vi "Advanced Generate LV Icon.vi"() -> ()   [LabVIEW 2020, in "LabVIEW Icon API.lvlib"]
doc: "This example shows an advanced way of using the LabVIEW Icon API."
uses:
  LabVIEW Icon API.lvlib
  lv_icon/Classes/Icon/Icon.lvclass
  API_Rectangle Dimension.ctl
  API_Text.ctl
  <vilib>/picture/picture.llb/imagedata.ctl
  <vilib>/Utility/miscctls.llb/LVPoint32TypeDef.ctl
  API_User Layer Data.ctl
  <vilib>/Utility/miscctls.llb/LVRectTypeDef.ctl
  API_Rectangle Colors.ctl
panel:
  out "Library Icon applied VI Icon":picture
  out "Updated VI Icon":picture
  out "Original VI Icon":picture
  out "Updated Library Icon":picture
  out "Original Library Icon":picture
  in  "Layer name":string="Circle"
  out "error out":errorcluster
  in  "error in (no error)":errorcluster
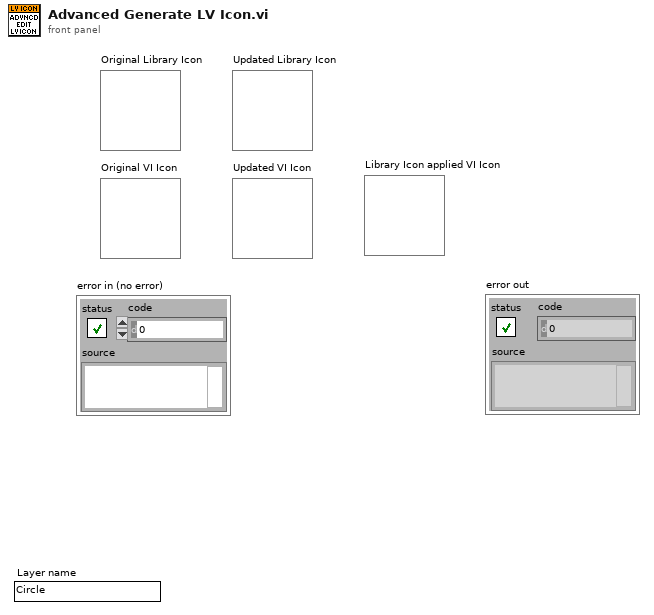
[diagram p1: front panel]
types:
  T1 = typedef "LabVIEW Icon API.lvlib/API_Rectangle Colors.ctl" = cluster{"Border":u32, "Background":u32}
  T2 = typedef "LVRectTypeDef.ctl" = cluster{"Left":i16, "Top":i16, "Right":i16, "Bottom":i16}
  T3 = cluster{"left":i16, "top":i16, "right":i16, "bottom":i16}
  T4 = typedef "LabVIEW Icon API.lvlib/API_User Layer Data.ctl" = cluster{"Layer name":string, "Origin":T5, "Icon image data":T6}
  T5 = typedef "LVPoint32TypeDef.ctl" = cluster{"Horizontal":i32, "Vertical":i32}
  T6 = typedef "imagedata.ctl" = cluster{"image type":i32, "image depth":i32, "image":u8[], "mask":u8[], "colors":u32[], "Rectangle":cluster{"left":i16, "top":i16, "right":i16, "bottom":i16}}
  T7 = typedef "LabVIEW Icon API.lvlib/API_Text.ctl" = cluster{"Line 1 text":string, "Line 2 text":string, "Line 3 text":string, "Line 4 text":string}
  T8 = typedef "LabVIEW Icon API.lvlib/API_Rectangle Dimension.ctl" = cluster{"Width":i16, "Height":i16}
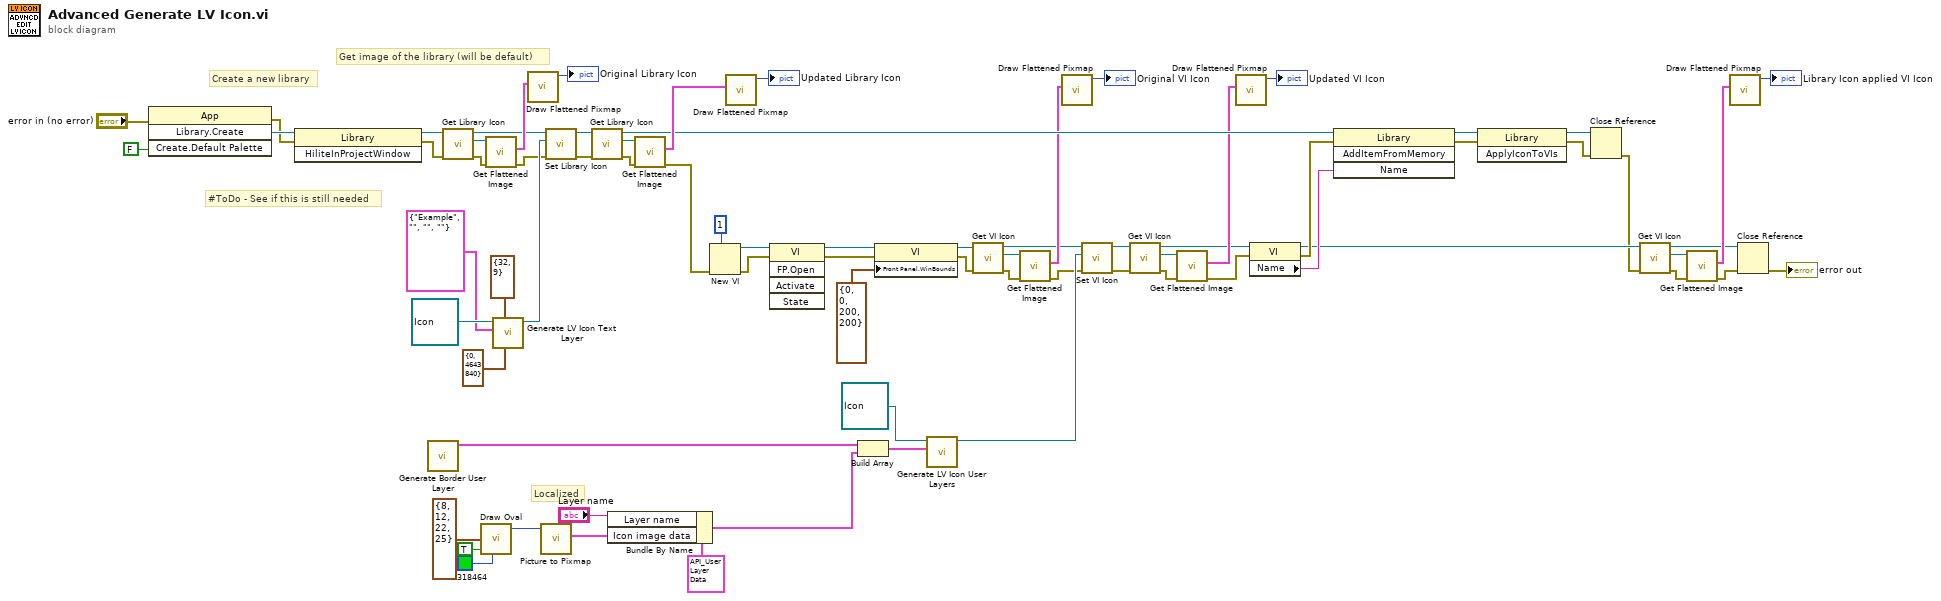
[diagram p0: block diagram]
diagram:
  # "#ToDo - See if this is still needed"
  # "Create a new library"
  # "Get image of the library (will be default)"
  # "Localized"
  n1 = invoke class="App" method="Library.Create"(error in="error in (no error)", "Create.Default Palette"=FALSE ("Create:Default Palette")) -> (error out=w67:errorcluster, "Create Library"=w68:refnum<vi>)  [unwired: 2 in, 2 out]
  n2 = invoke class="Library" method="HiliteInProjectWindow"(reference=w68, error in=w67) -> (reference out=w44:refnum<vi>, error out=w43:errorcluster)  [unwired: 1 in, 1 out]
  n3 = call "Generate Border User Layer.vi"() -> ("User Layer data"=w59:T4)  [unwired: 11 in]
  n4 = call "Get Library Icon.vi"("error in (no error)"=w43, "Library Refnum in"=w44) -> ("error out"=w41:errorcluster, "Icon"=w42:refnum<class "Icon.lvclass">, "Library Refnum out"=w38:refnum<vi>)  [unwired: 7 in]
  n5 = call <vilib>:"Draw Oval.vi"("rect"=T3 {"left"=8, "top"=12, "right"=22, "bottom"=25}, "fill?(F)"=TRUE, "color(black)"=u32 318464) -> ("new picture"=w63:picture)  [unwired: 6 in]
  n6 = call "Get Flattened Image.vi"("error in"=w41, "lv_icon.lvlib:Icon.lvclass in"=w42) -> ("error out"=w37:errorcluster, "Color Image"=w40:T6)  [unwired: 6 in, 2 out]
  n7 = call "Generate LV Icon Text Layer.vi"("Rectangle colors (black, white)"=T1 {"Border"=0, "Background"=4643840}, "Rectangle dimension (32,32)"=T8 {"Width"=32, "Height"=9}, "Text"=T7 {"Line 1 text"="Example", "Line 2 text"="", "Line 3 text"="", "Line 4 text"=""}, "Icon in"=refnum<class "Icon.lvclass"> refnum ("Icon.lvclass in")) -> ("Icon out"=w69:refnum<class "Icon.lvclass">)  [unwired: 6 in, 1 out]
  n8 = call <vilib>:"Draw Flattened Pixmap.vi"("image data"=w40) -> ("new picture"=→"Original Library Icon":picture)  [unwired: 8 in]
  n9 = call <vilib>:"Picture to Pixmap.vi"("picture"=w63) -> ("image data"=w61:T6)  [unwired: 9 in, 1 out]
  n10 = call "Set Library Icon.vi"("error in (no error)"=w37, "Icon"=w69, "Library Refnum in"=w38) -> ("error out"=w32:errorcluster, "Library Refnum out"=w31:refnum<vi>)  [unwired: 7 in]
  n11 = call "Get Library Icon.vi"("error in (no error)"=w32, "Library Refnum in"=w31) -> ("error out"=w34:errorcluster, "Icon"=w33:refnum<class "Icon.lvclass">, "Library Refnum out"=w30:refnum<vi>)  [unwired: 7 in]
  n12 = Bundle By Name(cluster=T4 {"Layer name"="", "Origin"={"Horizontal"=0, "Vertical"=0}, "Icon image data"={"image type"=0, "image depth"=0, "image"=[], "mask"=[], "colors"=[], "Rectangle"={"left"=0, "top"=0, "right"=0, "bottom"=0}}} ("User layer"), "Layer name"="Layer name", "Icon image data"=w61) -> (w58:T4)
  n13 = call "Get Flattened Image.vi"("error in"=w34, "lv_icon.lvlib:Icon.lvclass in"=w33) -> ("error out"=w29:errorcluster, "Color Image"=w35:T6)  [unwired: 6 in, 2 out]
  n14 = New VI(7:u32 1 ("options"), 8:w29) -> (0:w57:errorcluster, 3:w52:refnum<vi>)  [unwired: 5 in]
  n15 = call <vilib>:"Draw Flattened Pixmap.vi"("image data"=w35) -> ("new picture"=→"Updated Library Icon":picture)  [unwired: 8 in]
  n16 = invoke class="VI" method="FP.Open"(reference=w52, error in=w57) -> (reference out=w56:refnum<vi>, error out=w55:errorcluster)  [unwired: 3 in, 3 out]
  n17 = Build Array(w59, w58) -> (w51:T4[])
  n18 = property class="VI"(reference=w56, error in=w55, "Front Panel.WinBounds"=T2 {"Left"=0, "Top"=0, "Right"=200, "Bottom"=200} ("Front Panel Window:Window Bounds")) -> (reference out=w25:refnum<vi>, error out=w26:errorcluster)
  n19 = call "Generate LV Icon User Layers.vi"("User layers"=w51, "Icon in"=refnum<class "Icon.lvclass"> refnum) -> ("Icon out"=w49:refnum<class "Icon.lvclass">)  [unwired: 8 in, 1 out]
  n20 = call "Get VI Icon.vi"("error in (no error)"=w26, "VI Refnum in"=w25) -> ("error out"=w23:errorcluster, "Icon"=w24:refnum<class "Icon.lvclass">, "VI Refnum out"=w22:refnum<vi>)  [unwired: 7 in]
  n21 = call "Get Flattened Image.vi"("error in"=w23, "lv_icon.lvlib:Icon.lvclass in"=w24) -> ("error out"=w21:errorcluster, "Color Image"=w28:T6)  [unwired: 6 in, 2 out]
  n22 = call <vilib>:"Draw Flattened Pixmap.vi"("image data"=w28) -> ("new picture"=→"Original VI Icon":picture)  [unwired: 8 in]
  n23 = call "Set VI Icon.vi"("error in (no error)"=w21, "Icon"=w49, "VI Refnum in"=w22) -> ("error out"=w16:errorcluster, "VI Refnum out"=w17:refnum<vi>)  [unwired: 7 in]
  n24 = call "Get VI Icon.vi"("error in (no error)"=w16, "VI Refnum in"=w17) -> ("error out"=w20:errorcluster, "Icon"=w19:refnum<class "Icon.lvclass">, "VI Refnum out"=w14:refnum<vi>)  [unwired: 7 in]
  n25 = call "Get Flattened Image.vi"("error in"=w20, "lv_icon.lvlib:Icon.lvclass in"=w19) -> ("error out"=w13:errorcluster, "Color Image"=w18:T6)  [unwired: 6 in, 2 out]
  n26 = call <vilib>:"Draw Flattened Pixmap.vi"("image data"=w18) -> ("new picture"=→"Updated VI Icon":picture)  [unwired: 8 in]
  n27 = property class="VI"(reference=w14, error in=w13) -> (reference out=w9:refnum<vi>, error out=w47:errorcluster, "Name"=w48:string)
  n28 = invoke class="Library" method="AddItemFromMemory"(reference=w30, error in=w47, "Name"=w48) -> (reference out=w46:refnum<vi>, error out=w45:errorcluster)  [unwired: 1 in, 2 out]
  n29 = invoke class="Library" method="ApplyIconToVIs"(reference=w46, error in=w45) -> (reference out=w7:refnum<vi>, error out=w5:errorcluster)  [unwired: 1 in, 1 out]
  n30 = Close Reference(reference=w7, error in (no error)=w5) -> (error out=w4:errorcluster)
  n31 = call "Get VI Icon.vi"("error in (no error)"=w4, "VI Refnum in"=w9) -> ("error out"=w10:errorcluster, "Icon"=w11:refnum<class "Icon.lvclass">, "VI Refnum out"=w6:refnum<vi>)  [unwired: 7 in]
  n32 = call "Get Flattened Image.vi"("error in"=w10, "lv_icon.lvlib:Icon.lvclass in"=w11) -> ("error out"=w3:errorcluster, "Color Image"=w8:T6)  [unwired: 6 in, 2 out]
  n33 = call <vilib>:"Draw Flattened Pixmap.vi"("image data"=w8) -> ("new picture"=→"Library Icon applied VI Icon":picture)  [unwired: 8 in]
  n34 = Close Reference(reference=w6, error in (no error)=w3) -> (error out=→"error out":errorcluster)
